vi "Change Constants VI.vi"(4 "Extra Page GUIDs":string[](array[string]), 6 "Extra Page Names":string[](array[string]), 7 "CD Template":refnum<class "NIVS_CD Template.lvclass">, 8 "error in (no error)":errorcluster, 9 "Constants.vi path":path, 10 "CD GUID":string, 11 "CD Name":string) -> (0 "error out":errorcluster)   [LabVIEW 2017, in "NIVS_Consolidated_CDW_MetaDataObj.lvclass"]
doc: "This VI alters the frontpanel of the <B>Constants.VI template</B>. It adds a control for each extra page and the custom device itself to the frontpanel. The control is labeled according to the name of the custom device/extra page and contains the GUID for the corresponding object."
uses:
  NIVS_Consolidated_CDW_MetaDataObj.lvclass
  Template Classes/NIVS_CD Template/NIVS_CD Template.lvclass
  Extra Page Name and GUID.ctl
  <vilib>/Utility/miscctls.llb/LVBoundsTypeDef.ctl
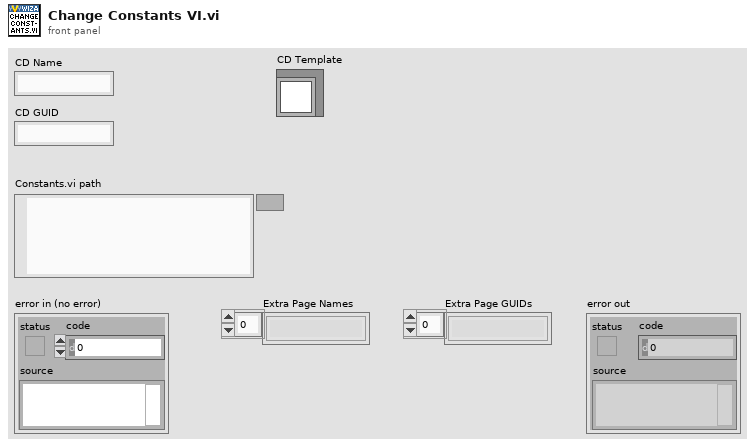
[diagram p1: front panel]
types:
  T1 = typedef "LVBoundsTypeDef.ctl" = cluster{"Width":u32, "Height":u32}
  T2 = typedef "NIVS_Consolidated_CDW_MetaDataObj.lvclass/Extra Page Name and GUID.ctl" = cluster{"Page Name":string, "Page GUID":string}
  T3 = typedef "NIVS_Consolidated_CDW_MetaDataObj.lvclass/Property Information.ctl" = cluster{"Name":string, "Value":variant, "Type":string}
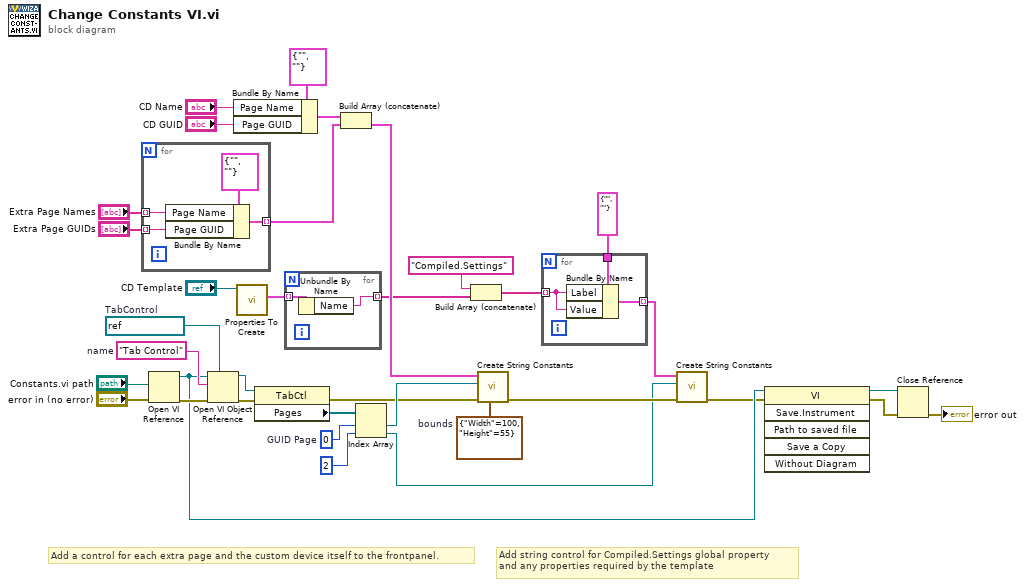
[diagram p0: block diagram]
diagram:
  w12 = T1 {"Width"=100, "Height"=55}  # bounds
  w32 = 0  # GUID Page
  w30 = refnum<vi> refnum  # TabControl
  w29 = "Tab Control"  # name
  # "Add a control for each extra page and the custom device itself to the frontpanel."
  # "Add string control for Compiled.Settings global property\nand any properties required by the template"
  n1 = for {
    tunnel: "Extra Page Names" -> [w38] mode=indexing
    tunnel: "Extra Page GUIDs" -> [w37] mode=indexing
    tunnel: [w36] -> w15 mode=indexing
    n2 = Bundle By Name(cluster=T2 {"Page Name"="", "Page GUID"=""} ("Extra Page"), "Page Name"=w38, "Page GUID"=w37) -> (w36:T2)
  }
  n3 = Open VI Reference(vi path="Constants.vi path", error in (no error)="error in (no error)") -> (vi reference=w27:refnum<vi>, error out=w28:errorcluster)  [unwired: 4 in]
  n4 = Open VI Object Reference(7:w30, 8:w28, 10:w29, 11:w27) -> (0:w31:errorcluster, 3:w26:refnum<vi>)
  n5 = Bundle By Name(cluster=T2 {"Page Name"="", "Page GUID"=""} ("Extra Page"), "Page Name"="CD Name", "Page GUID"="CD GUID") -> (w21:T2)
  n6 = call-dynamic "Properties To Create.vi"("CD Template in"="CD Template") -> ("Properties"=w2:T3[])  [unwired: 9 in, 1 out]
  n7 = property class="TabCtl"(reference=w26, error in=w31) -> (error out=w11:errorcluster, "Pages"=w25:refnum<vi>[])  [unwired: 1 out]
  n8 = for {
    tunnel: w2 -> [w41] mode=indexing
    tunnel: [w40] -> w1 mode=indexing
    n9 = Unbundle By Name(w41) -> ("Name"=w40:string)
  }
  n10 = Build Array (concatenate)(w21, w15) -> (w14:T2[])
  n11 = Index Array(array=w25, index #1=w32, index #2=2 ("index")) -> (element #1=w13:refnum<vi>, element #2=w9:refnum<vi>)
  n12 = Build Array (concatenate)("Compiled.Settings" ("Page Name"), w1) -> (w6:string[])
  n13 = call "Create String Constants.vi"("bounds"=w12, "error in (no error)"=w11, "Page Refnum"=w13, "Constants"=w14) -> ("error out"=w10:errorcluster)  [unwired: 7 in]
  n14 = for {
    tunnel: w6 -> [w44] mode=indexing
    tunnel: [w43] -> w4 mode=indexing
    tunnel: cluster{"Label":string, "Value":string} {"Label"="", "Value"=""} ("Constant") -> [w42]
    n15 = Bundle By Name(cluster=w42, "Label"=w44, "Value"=w44) -> (w43:cluster{"Label":string, "Value":string})
  }
  n16 = call "Create String Constants.vi"("error in (no error)"=w10, "Page Refnum"=w9, "Constants"=w4) -> ("error out"=w3:errorcluster)  [unwired: 8 in]
  n17 = invoke class="VI" method="Save.Instrument"(reference=w27, error in=w3) -> (reference out=w24:refnum<vi>, error out=w23:errorcluster)  [unwired: 4 in, 4 out]
  n18 = Close Reference(reference=w24, error in (no error)=w23) -> (error out=→"error out":errorcluster)
